vi "string_defaultvalue.vi"() -> ()   [LabVIEW 2020]
panel:
  in  "string":string="a\nb\nc"
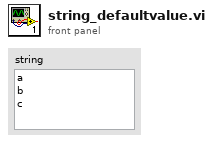
[diagram p1: front panel]
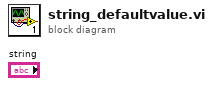
[diagram p0: block diagram]
diagram:
